vi "GetColorStyle.vi"(1 "ColorStyle":T1(ring)) -> (0 "FalseColorData":T2)   [LabVIEW 2016]
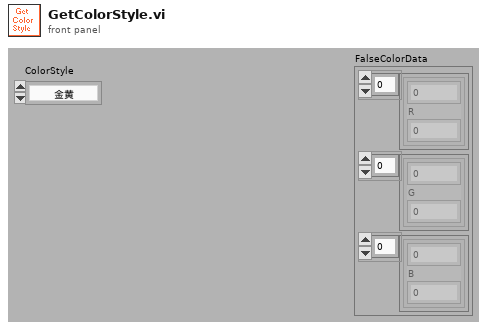
[diagram p1: front panel]
types:
  T1 = enum16{"金黄", "墨绿", "草绿", "蓝色", "紫色", "棕色", "灰度", "高对比", "反白"}
  T2 = cluster{cluster{dbl, "R":dbl}[], cluster{dbl, "G":dbl}[], cluster{dbl, "B":dbl}[]}
  T3 = cluster{cluster{"y":dbl, "R":dbl}[], cluster{"y":dbl, "R":dbl}[], cluster{"y":dbl, "R":dbl}[]}
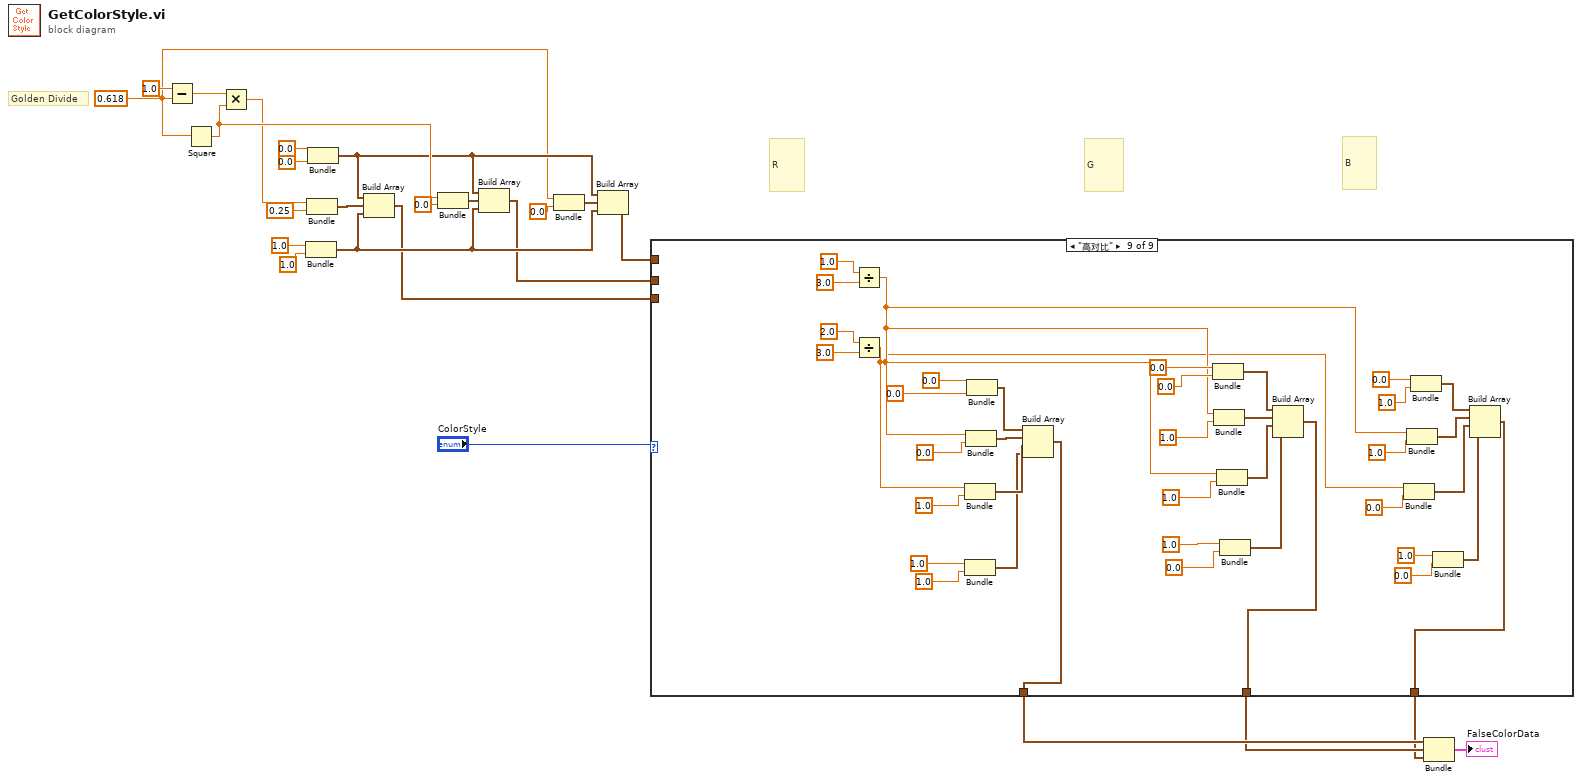
[diagram p0: block diagram]
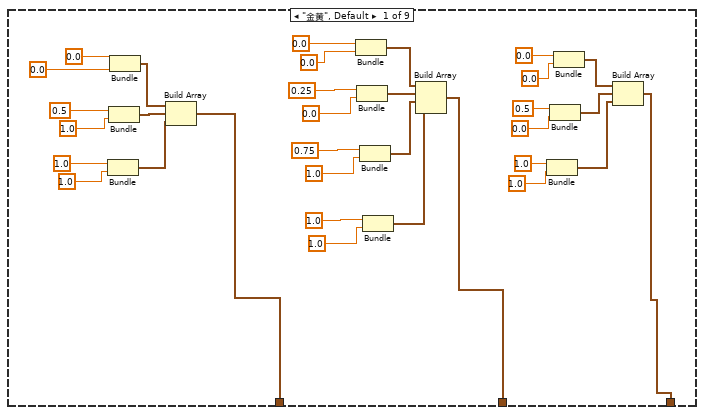
[diagram p2: hidden frame]
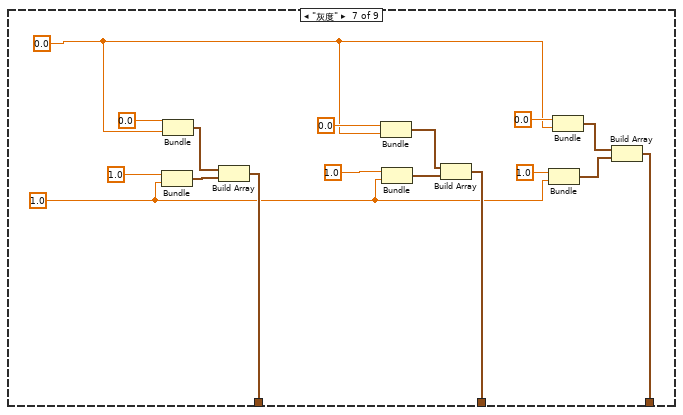
[diagram p8: hidden frame]
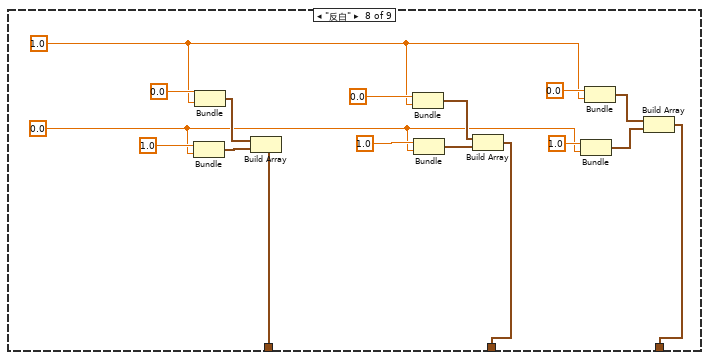
[diagram p9: hidden frame]
diagram:
  w1 = 0.618 ("y")
  # "Golden Divide"
  # "B"
  # "G"
  # "R"
  n1 = Subtract(x=1.0, y=w1) -> (x-y=w11:dbl)
  n2 = Square(x=w1) -> (x^2=w8:dbl)
  n3 = Multiply(x=w11, y=w8) -> (x*y=w2:dbl)
  n4 = Bundle(1.0, "R"=1.0) -> (w7:cluster{dbl, "R":dbl})  [unwired: 1 out]
  n5 = Bundle(w2, "R"=0.25) -> (w15:cluster{dbl, "R":dbl})  [unwired: 1 out]
  n6 = Bundle(0.0, "R"=0.0) -> (w6:cluster{dbl, "R":dbl})  [unwired: 1 out]
  n7 = Build Array(w6, w15, w7) -> (w5:cluster{dbl, "R":dbl}[])
  n8 = Bundle(w8, "R"=0.0) -> (w13:cluster{dbl, "R":dbl})  [unwired: 1 out]
  n9 = Build Array(w6, w13, w7) -> (w4:cluster{dbl, "R":dbl}[])
  n10 = Bundle("y"=w1, "R"=0.0) -> (w10:cluster{"y":dbl, "R":dbl})  [unwired: 1 out]
  n11 = Build Array(w6, w10, w7) -> (w3:cluster{"y":dbl, "R":dbl}[])
  n12 = case shown="\"高对比\"" "ColorStyle" {
    tunnel: [w31 w59 w63 w65 w70 w73 w78 w95 w115] -> w25
    tunnel: [w30 w60 w64 w67 w68 w72 w77 w94 w110] -> w24
    tunnel: [w29 w61 w62 w66 w69 w71 w76 w93 w109] -> w23
    tunnel: w5 -> [_ w60 w64 w66 w69 w73 _ _ _]
    tunnel: w4 -> [_ w61 w63 w67 w70 w72 _ _ _]
    tunnel: w3 -> [_ w59 w62 w65 w68 w71 _ _ _]
    frame "金黄", Default {
      n13 = Bundle(1.0, "R"=1.0) -> (w43:cluster{dbl, "R":dbl})  [unwired: 1 out]
      n14 = Bundle(0.5, "R"=1.0) -> (w58:cluster{dbl, "R":dbl})  [unwired: 1 out]
      n15 = Bundle(0.0, "R"=0.0) -> (w57:cluster{dbl, "R":dbl})  [unwired: 1 out]
      n16 = Build Array(w57, w58, w43) -> (w31:cluster{dbl, "R":dbl}[])
      n17 = Bundle(0.0, "R"=0.0) -> (w52:cluster{dbl, "R":dbl})  [unwired: 1 out]
      n18 = Bundle(0.25, "R"=0.0) -> (w51:cluster{dbl, "R":dbl})  [unwired: 1 out]
      n19 = Bundle(0.75, "R"=1.0) -> (w37:cluster{dbl, "R":dbl})  [unwired: 1 out]
      n20 = Bundle(1.0, "R"=1.0) -> (w26:cluster{dbl, "R":dbl})  [unwired: 1 out]
      n21 = Build Array(w52, w51, w37, w26) -> (w30:cluster{dbl, "R":dbl}[])
      n22 = Bundle(1.0, "R"=1.0) -> (w32:cluster{dbl, "R":dbl})  [unwired: 1 out]
      n23 = Bundle(0.5, "R"=0.0) -> (w50:cluster{dbl, "R":dbl})  [unwired: 1 out]
      n24 = Bundle(0.0, "R"=0.0) -> (w49:cluster{dbl, "R":dbl})  [unwired: 1 out]
      n25 = Build Array(w49, w50, w32) -> (w29:cluster{dbl, "R":dbl}[])
    }
    frame "墨绿" {
    }
    frame "草绿" {
    }
    frame "蓝色" {
    }
    frame "紫色" {
    }
    frame "棕色" {
    }
    frame "灰度" {
      w74 = 0.0 ("B")
      w75 = 1.0 ("B")
      n26 = Bundle(1.0, "B"=w75) -> (w90:cluster{dbl, "B":dbl})  [unwired: 1 out]
      n27 = Bundle(0.0, "B"=w74) -> (w89:cluster{dbl, "B":dbl})  [unwired: 1 out]
      n28 = Build Array(w89, w90) -> (w78:cluster{dbl, "B":dbl}[])
      n29 = Bundle(0.0, "B"=w74) -> (w84:cluster{dbl, "B":dbl})  [unwired: 1 out]
      n30 = Bundle(1.0, "B"=w75) -> (w83:cluster{dbl, "B":dbl})  [unwired: 1 out]
      n31 = Build Array(w84, w83) -> (w77:cluster{dbl, "B":dbl}[])
      n32 = Bundle(1.0, "B"=w75) -> (w82:cluster{dbl, "B":dbl})  [unwired: 1 out]
      n33 = Bundle(0.0, "B"=w74) -> (w81:cluster{dbl, "B":dbl})  [unwired: 1 out]
      n34 = Build Array(w81, w82) -> (w76:cluster{dbl, "B":dbl}[])
    }
    frame "反白" {
      w91 = 0.0
      w92 = 1.0
      n35 = Bundle(1.0, w91) -> (w107:cluster{dbl, dbl})  [unwired: 1 out]
      n36 = Bundle(0.0, w92) -> (w106:cluster{dbl, dbl})  [unwired: 1 out]
      n37 = Build Array(w106, w107) -> (w95:cluster{dbl, dbl}[])
      n38 = Bundle(0.0, w92) -> (w101:cluster{dbl, dbl})  [unwired: 1 out]
      n39 = Bundle(1.0, w91) -> (w100:cluster{dbl, dbl})  [unwired: 1 out]
      n40 = Build Array(w101, w100) -> (w94:cluster{dbl, dbl}[])
      n41 = Bundle(1.0, w91) -> (w99:cluster{dbl, dbl})  [unwired: 1 out]
      n42 = Bundle(0.0, w92) -> (w98:cluster{dbl, dbl})  [unwired: 1 out]
      n43 = Build Array(w98, w99) -> (w93:cluster{dbl, dbl}[])
    }
    frame "高对比" {
      n44 = Divide(x=1.0, y=3.0) -> (x/y=w114:dbl)
      n45 = Divide(x=2.0, y=3.0) -> (x/y=w113:dbl)
      n46 = Bundle(w113, "R"=1.0) -> (w135:cluster{dbl, "R":dbl})  [unwired: 1 out]
      n47 = Bundle(1.0, "R"=1.0) -> (w116:cluster{dbl, "R":dbl})  [unwired: 1 out]
      n48 = Bundle(w114, "R"=0.0) -> (w146:cluster{dbl, "R":dbl})  [unwired: 1 out]
      n49 = Bundle(0.0, "R"=0.0) -> (w145:cluster{dbl, "R":dbl})  [unwired: 1 out]
      n50 = Build Array(w145, w146, w135, w116) -> (w115:cluster{dbl, "R":dbl}[])
      n51 = Bundle(0.0, "R"=0.0) -> (w142:cluster{dbl, "R":dbl})  [unwired: 1 out]
      n52 = Bundle(w114, "R"=1.0) -> (w141:cluster{dbl, "R":dbl})  [unwired: 1 out]
      n53 = Bundle(w113, "R"=1.0) -> (w130:cluster{dbl, "R":dbl})  [unwired: 1 out]
      n54 = Bundle(1.0, "R"=0.0) -> (w123:cluster{dbl, "R":dbl})  [unwired: 1 out]
      n55 = Build Array(w142, w141, w130, w123) -> (w110:cluster{dbl, "R":dbl}[])
      n56 = Bundle(w113, "R"=0.0) -> (w126:cluster{dbl, "R":dbl})  [unwired: 1 out]
      n57 = Bundle(w114, "R"=1.0) -> (w140:cluster{dbl, "R":dbl})  [unwired: 1 out]
      n58 = Bundle(0.0, "R"=1.0) -> (w139:cluster{dbl, "R":dbl})  [unwired: 1 out]
      n59 = Bundle(1.0, "R"=0.0) -> (w108:cluster{dbl, "R":dbl})  [unwired: 1 out]
      n60 = Build Array(w139, w140, w126, w108) -> (w109:cluster{dbl, "R":dbl}[])
    }
  }
  n61 = Bundle(w25, w24, w23) -> (→"FalseColorData":T3)  [unwired: 1 out]
